vi "MainScriptCreateAllIOselectors.vi"   [LabVIEW 2024]
uses:
  <vilib>/numeric/LVNumericRepresentation.ctl
panel:
  # "VI for creating by scripting all the FPGA I/O node selectors,\nbased on case structures wrapping individual Element I/Os"
types:
  T1 = typedef "LVNumericRepresentation.ctl" = enum32{"Extended Precision", "Double Precision", "Single Precision", "Long", "Word", "Byte", "Unsigned Long", "Unsigned Word", "Unsigned Byte", "Complex Extended", "Complex Double", "Complex Single", "Quad", "Unsigned Quad", "Fixed-Point"}
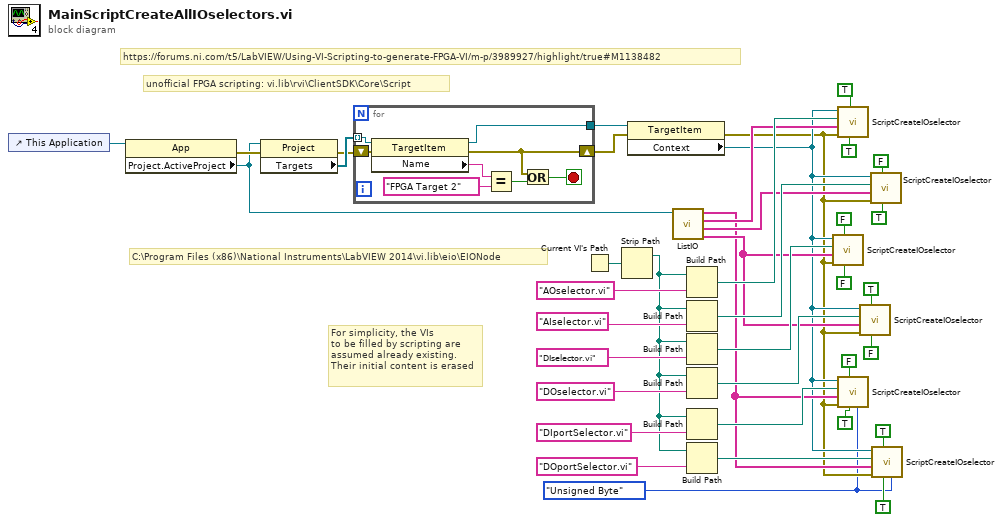
[diagram p0: block diagram]
diagram:
  w1 = LVNumericRepresentation."Unsigned Byte" ("numeric representation")
  # "For simplicity, the VIs\nto be filled by scripting are\nassumed already existing.\nTheir initial content is erased"
  # "C:\\Program Files (x86)\\National Instruments\\LabVIEW 2014\\vi.lib\\eio\\EIONode"
  # "https://forums.ni.com/t5/LabVIEW/Using-VI-Scripting-to-generate-FPGA-VI/m-p/3989927/highlight/true#M1138482"
  # "unofficial FPGA scripting: vi.lib\\rvi\\ClientSDK\\Core\\Script"
  n1 = control-ref of="This Application"() -> (w33:refnum<vi>)
  n2 = property class="App"(reference=w33) -> (error out=w36:errorcluster, "Project.ActiveProject"=w18:refnum<vi>)  [unwired: 1 in, 1 out]
  n3 = property class="Project"(reference=w18, error in=w36) -> (error out=w35:errorcluster, "Targets"=w40:refnum<vi>[])  [unwired: 1 out]
  n4 = for {
    tunnel: w40 -> [w48] mode=indexing
    tunnel: [w45] -> w37
    shift-right: [w41] -> w34
    shift-left: w35 -> [w43]
    stop <- w42 stop-if-true
    n5 = property class="TargetItem"(reference=w48, error in=w43) -> (reference out=w45:refnum<vi>, error out=w41:errorcluster, "Name"=w47:string)
    n6 = Equal?(x=w47, y="FPGA Target 2" ("String")) -> (x = y?=w46:bool)
    n7 = Or(x=w41, y=w46) -> (x .or. y?=w42:bool)
  }
  n8 = Current VI's Path() -> (path=w39:path)
  n9 = Strip Path(path=w39) -> (stripped path=w2:path)  [unwired: 1 out]
  n10 = property class="TargetItem"(reference=w37, error in=w34) -> (error out=w3:errorcluster, "Context"=w4:refnum<vi>)  [unwired: 1 out]
  n11 = call "ListIO.vi"("Project"=w18) -> ("DI/O"=w13:string[], "AI"=w16:string[], "AO"=w17:string[], "DIOPORT"=w5:string[])  [unwired: 6 in, 1 out]
  n12 = Build Path(base path=w2, name or relative path="AOselector.vi") -> (appended path=w31:path)
  n13 = Build Path(base path=w2, name or relative path="AIselector.vi") -> (appended path=w21:path)
  n14 = Build Path(base path=w2, name or relative path="DIselector.vi") -> (appended path=w24:path)
  n15 = Build Path(base path=w2, name or relative path="DOselector.vi") -> (appended path=w25:path)
  n16 = Build Path(base path=w2, name or relative path="DIportSelector.vi") -> (appended path=w8:path)
  n17 = Build Path(base path=w2, name or relative path="DOportSelector.vi") -> (appended path=w7:path)
  n18 = call "ScriptCreateIOselector.vi"("digital(F)/numeric(T)"=FALSE, "indicator (F)/control (T)"=FALSE, "error in (no error)"=w3, "IO names"=w13, "VI path"=w24, "Application in"=w4) -> ()  [unwired: 6 in]
  n19 = call "ScriptCreateIOselector.vi"("digital(F)/numeric(T)"=TRUE, "indicator (F)/control (T)"=TRUE, "error in (no error)"=w3, "IO names"=w17, "VI path"=w31, "Application in"=w4) -> ()  [unwired: 6 in]
  n20 = call "ScriptCreateIOselector.vi"("numeric representation"=w1, "digital(F)/numeric(T)"=TRUE, "indicator (F)/control (T)"=FALSE, "error in (no error)"=w3, "IO names"=w5, "VI path"=w8, "Application in"=w4) -> ()  [unwired: 5 in]
  n21 = call "ScriptCreateIOselector.vi"("digital(F)/numeric(T)"=FALSE, "indicator (F)/control (T)"=TRUE, "error in (no error)"=w3, "IO names"=w13, "VI path"=w25, "Application in"=w4) -> ()  [unwired: 6 in]
  n22 = call "ScriptCreateIOselector.vi"("digital(F)/numeric(T)"=TRUE, "indicator (F)/control (T)"=FALSE, "error in (no error)"=w3, "IO names"=w16, "VI path"=w21, "Application in"=w4) -> ()  [unwired: 6 in]
  n23 = call "ScriptCreateIOselector.vi"("numeric representation"=w1, "digital(F)/numeric(T)"=TRUE, "indicator (F)/control (T)"=TRUE, "error in (no error)"=w3, "IO names"=w5, "VI path"=w7, "Application in"=w4) -> ()  [unwired: 5 in]
